vi "Compile Settings.vi"(8 "error in":errorcluster, 10 "Settings(JSON)":string, 11 "Custom Device Deployment Hooks in":refnum<class "NIDMM Deployment Hooks.lvclass">) -> (0 "error out":errorcluster, 2 "Compiled Settings":variant, 3 "Custom Device Deployment Hooks out":refnum<class "NIDMM Deployment Hooks.lvclass">)   [LabVIEW 2026, in "NIDMM Deployment Hooks.lvlib" / "NIDMM Deployment Hooks.lvclass"]
uses:
  NIDMM Deployment Hooks.lvclass
  NIDMM Deployment Hooks.lvclass/NIDMM Deployment Hooks.ctl
  <vilib>/JDP Science/JSONtext/JSONtext.lvlib
  NIDMM Deployment Hooks.lvlib
  Shared/CustomDeviceSettings.ctl
  Shared/GroupedChannelRefs.ctl
  Shared/GroupedChannel.ctl
  Shared/GroupSettings.ctl
  Shared/ChannelGroups.ctl
  Shared/Compiled.Settings.ctl
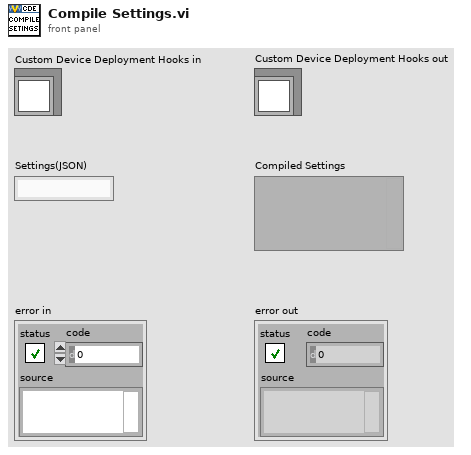
[diagram p1: front panel]
types:
  T1 = typedef "Compiled.Settings.ctl" = cluster{"NIDMM":T2, "Channel Groups":T3}
  T2 = typedef "CustomDeviceSettings.ctl" = cluster{"Name":string, "Properties":cluster{"ResourceName":string, "Model":string, "ScanPeriod(ms)":dbl, "ResolutionDigits":dbl, "ACMaxFrequency":dbl, "ACMinFrequency":dbl, "TargetOS":string, "TargetRate":dbl}, "Channels":cluster{"Mode[]":cluster{"Name":string, "DefaultValue":dbl, "Units":string, "GroupName":string, "Type":string, "Faultable":bool, "Scalable":bool, "ChannelDataReference":i32, "GroupIndex":i32}[], "ActiveMode[]":cluster{"Name":string, "DefaultValue":dbl, "Units":string, "GroupName":string, "Type":string, "Faultable":bool, "Scalable":bool, "ChannelDataReference":i32, "GroupIndex":i32}[], "DeviceStatus[]":cluster{"Name":string, "DefaultValue":dbl, "Units":string, "GroupName":string, "Type":string, "Faultable":bool, "Scalable":bool, "ChannelDataReference":i32, "GroupIndex":i32}[], "Heartbeat[]":cluster{"Name":string, "DefaultValue":dbl, "Units":string, "GroupName":string, "Type":string, "Faultable":bool, "Scalable":bool, "ChannelDataReference":i32, "GroupIndex":i32}[]}, "Sections":cluster{"Voltage[]":cluster{"Name":string, "Channels":cluster{"VoltageReading[]":cluster{"Name":string, "DefaultValue":dbl, "Units":string, "GroupName":string, "Type":string, "Faultable":bool, "Scalable":bool, "ChannelDataReference":i32, "GroupIndex":i32}[], "VoltageStatus[]":cluster{"Name":string, "DefaultValue":dbl, "Units":string, "GroupName":string, "Type":string, "Faultable":bool, "Scalable":bool, "ChannelDataReference":i32, "GroupIndex":i32}[], "VoltageFunction[]":cluster{"Name":string, "DefaultValue":dbl, "Units":string, "GroupName":string, "Type":string, "Faultable":bool, "Scalable":bool, "ChannelDataReference":i32, "GroupIndex":i32}[], "VoltageActualRange[]":cluster{"Name":string, "DefaultValue":dbl, "Units":string, "GroupName":string, "Type":string, "Faultable":bool, "Scalable":bool, "ChannelDataReference":i32, "GroupIndex":i32}[], "VoltageRange[]":cluster{"Name":string, "DefaultValue":dbl, "Units":string, "GroupName":string, "Type":string, "Faultable":bool, "Scalable":bool, "ChannelDataReference":i32, "GroupIndex":i32}[]}}[], "Current[]":cluster{"Name":string, "Channels":cluster{"CurrentReading[]":cluster{"Name":string, "DefaultValue":dbl, "Units":string, "GroupName":string, "Type":string, "Faultable":bool, "Scalable":bool, "ChannelDataReference":i32, "GroupIndex":i32}[], "CurrentStatus[]":cluster{"Name":string, "DefaultValue":dbl, "Units":string, "GroupName":string, "Type":string, "Faultable":bool, "Scalable":bool, "ChannelDataReference":i32, "GroupIndex":i32}[], "CurrentFunction[]":cluster{"Name":string, "DefaultValue":dbl, "Units":string, "GroupName":string, "Type":string, "Faultable":bool, "Scalable":bool, "ChannelDataReference":i32, "GroupIndex":i32}[], "CurrentActualRange[]":cluster{"Name":string, "DefaultValue":dbl, "Units":string, "GroupName":string, "Type":string, "Faultable":bool, "Scalable":bool, "ChannelDataReference":i32, "GroupIndex":i32}[], "CurrentRange[]":cluster{"Name":string, "DefaultValue":dbl, "Units":string, "GroupName":string, "Type":string, "Faultable":bool, "Scalable":bool, "ChannelDataReference":i32, "GroupIndex":i32}[]}}[]}}
  T3 = typedef "ChannelGroups.ctl" = cluster{"Channel Refs":T4, "Group Settings":T5[]}
  T4 = typedef "GroupedChannelRefs.ctl" = cluster{"Read":cluster{"Refs":cluster{"Data Reference":i32, "Offset":u64, "Length":u64}[], "Values":dbl[]}[], "Write":cluster{"Refs":cluster{"Data Reference":i32, "Offset":u64, "Length":u64}[], "Values":dbl[]}[], "ReadWrite":cluster{"Refs":i32[], "Values":dbl[], "Reset Values":dbl[]}[], "LUT":variant}
  T5 = typedef "GroupSettings.ctl" = cluster{"Name":string, "Type":enum16{"Output/Write", "Input/Read", "Input/ReadWrite"}, "Channel Settings":T6[]}
  T6 = typedef "GroupedChannel.ctl" = cluster{"Name":string, "TypeName":string, "ChannelProperties":variant}
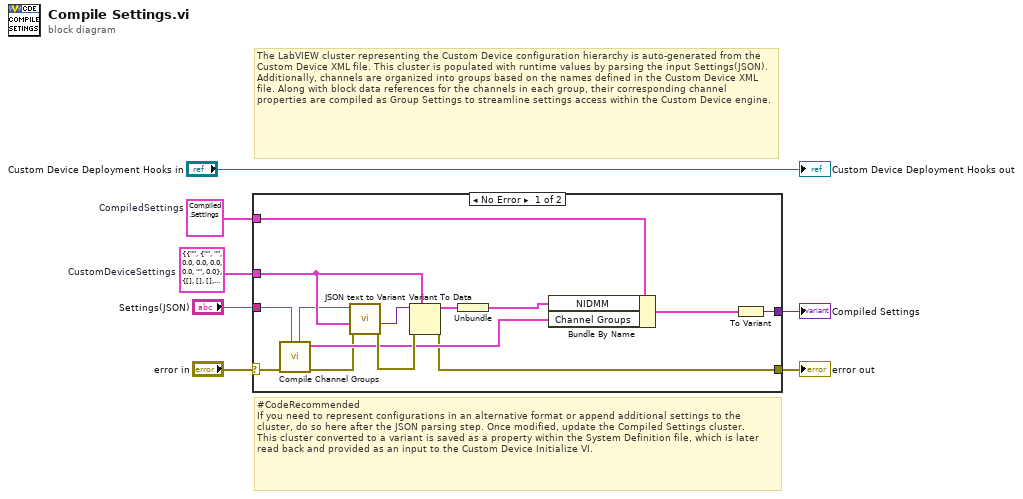
[diagram p0: block diagram]
diagram:
  w2 = T1 {"NIDMM"={"Name"="", "Properties"={"ResourceName"="", "Model"="", "ScanPeriod(ms)"=0.0, "ResolutionDigits"=0.0, "ACMaxFrequency"=0.0, "ACMinFrequency"=0.0, "TargetOS"="", "TargetRate"=0.0}, "Channels"={"Mode[]"=[], "ActiveMode[]"=[], "DeviceStatus[]"=[], "Heartbeat[]"=[]}, "Sections"={"Voltage[]"=[], "Current[]"=[]}}, "Channel Groups"={"Channel Refs"={"Read"=[], "Write"=[], "ReadWrite"=[], "LUT"=variant}, "Group Settings"=[]}}  # CompiledSettings
  w3 = cluster{"NIDMM":T2} {"NIDMM"={"Name"="", "Properties"={"ResourceName"="", "Model"="", "ScanPeriod(ms)"=0.0, "ResolutionDigits"=0.0, "ACMaxFrequency"=0.0, "ACMinFrequency"=0.0, "TargetOS"="", "TargetRate"=0.0}, "Channels"={"Mode[]"=[], "ActiveMode[]"=[], "DeviceStatus[]"=[], "Heartbeat[]"=[]}, "Sections"={"Voltage[]"=[], "Current[]"=[]}}}  # CustomDeviceSettings
  # "#CodeRecommended \nIf you need to represent configurations in an alternative format or append additional settings to the cluster, do so here after the JSON parsing step. Once modified, update the Compiled Settings cluster. \nThis cluster converted to a variant is saved as a property within the System Definition file, which is later read back and provided as an input to the Custom Device Initialize VI."
  # "The LabVIEW cluster representing the Custom Device configuration hierarchy is auto-generated from the Custom Device XML file. This cluster is populated with runtime values by parsing the input Settings(JSON). \nAdditionally, channels are organized into groups based on the names defined in the Custom Device XML file. Along with block data references for the channels in each group, their corresponding channel properties are compiled as Group Settings to streamline settings access within the Custom Device engine."
  n1 = case shown="No Error" "error in" {
    selector: "error in" -> [w11 w22]
    tunnel: "Settings(JSON)" -> [w13 _]
    tunnel: [w21 _] -> w4
    tunnel: [w9 w22] -> w6
    tunnel: w3 -> [w20 _]
    tunnel: w2 -> [w19 _]
    frame No Error {
      n2 = call "Compile Channel Groups.vi"("Settings(JSON)"=w13, "error in"=w11) -> ("error out"=w10:errorcluster, "ChannelGroups"=w14:T3, "Settings(JSON)"=w12:string)  [unwired: 7 in]
      n3 = call <vilib>:"JSON text to Variant.vi"("error in (no error)"=w10, "Data Type"=w20, "JSON"=w12) -> ("error out"=w18:errorcluster, "Variant out"=w17:variant)  [unwired: 7 in]
      n4 = Variant To Data(error in=w18, type=w20, Variant=w17) -> (data=w16:cluster{"NIDMM":T2}, error out=w9:errorcluster)
      n5 = Unbundle(w16) -> ("NIDMM"=w8:T2)
      n6 = Bundle By Name(cluster=w19, "NIDMM"=w8, "Channel Groups"=w14) -> (w15:T1)
      n7 = To Variant(anything=w15) -> (Variant=w21:variant)
    }
    frame Error {
    }
  }
  "error out" <- w6
  "Compiled Settings" <- w4
  "Custom Device Deployment Hooks out" <- "Custom Device Deployment Hooks in"
